vi "create scan vectr.vi"(2 "Table Control":string[][](table), 3 "waypoint mode?":bool=TRUE) -> (0 "Array 2":dbl[](array[numeric]), 1 "Array":dbl[](array[numeric]))   [LabVIEW 2020]
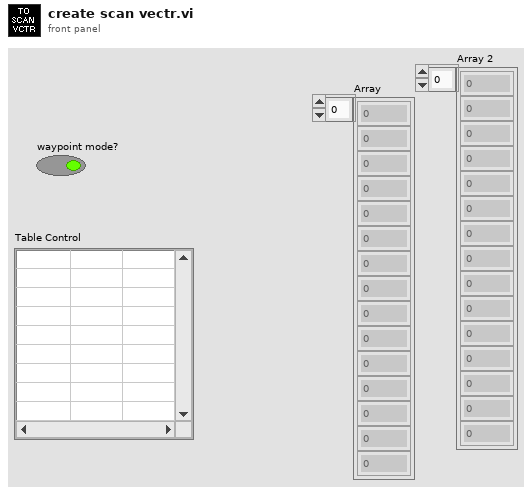
[diagram p1: front panel]
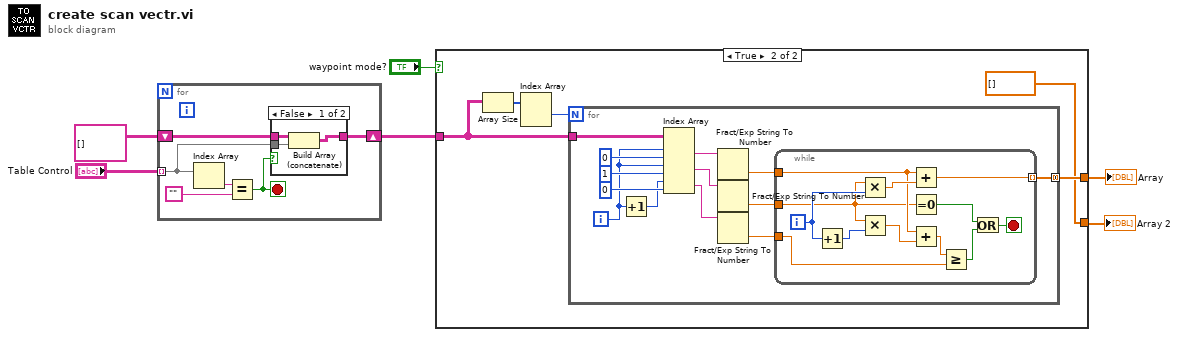
[diagram p0: block diagram]
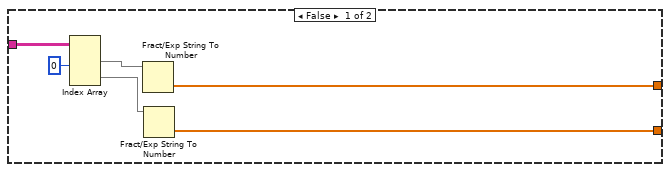
[diagram p2: hidden frame]
diagram:
  n1 = for {
    tunnel: "Table Control" -> [w8] mode=indexing
    shift-right: [w7] -> w3
    shift-left: string[][] [] ("t") -> [w10]
    stop <- w9 stop-if-true
    n2 = Index Array(array=w8) -> (element=w11:string)  [unwired: 1 in]
    n3 = Equal?(x=w11, y="") -> (x = y?=w9:bool)
    n4 = case shown="False" w9 {
      tunnel: w10 -> [w15 w16]
      tunnel: w8 -> [w14 _]
      tunnel: [w13 w16] -> w7
      frame False {
        n5 = Build Array (concatenate)(w15, w14) -> (w13:string[][])
      }
      frame True {
      }
    }
  }
  n6 = case shown="True" "waypoint mode?" {
    tunnel: [w20 w25] -> w4
    tunnel: w3 -> [w21 w24]
    tunnel: [w17 dbl[] []] -> w1
    frame False {
      n7 = Index Array(array=w21, index (col) #1=0 ("disabled index (col)")) -> (element #1=w22:string[], element #2=w18:string[])  [unwired: 3 in]
      n8 = Fract/Exp String To Number(string=w22) -> (number=w20:dbl[])  [unwired: 3 in, 1 out]
      n9 = Fract/Exp String To Number(string=w18) -> (number=w17:dbl[])  [unwired: 3 in, 1 out]
    }
    frame True {
      n10 = Array Size(array=w24) -> (size(s)=w27:i32[])
      n11 = Index Array(array=w27) -> (element #1=w26:i32)  [unwired: 2 in, 1 out]
      n12 = for {
        N: w26 -> [_]
        tunnel: w24 -> [w36]
        tunnel: [w28] -> w25 mode=concatenating
        i -> [w35]
        n13 = Increment(x=w35) -> (x+1=w38:i32)
        n14 = Index Array(array=w36, index (row) #1=w35, index (col) #1=0 ("disabled index (col)"), index (row) #2=w35, index (col) #2=1 ("disabled index (col)"), index (row) #3=w38, index (col) #3=0 ("disabled index (col)")) -> (element #1=w34:string, element #2=w33:string, element #3=w32:string)
        n15 = Fract/Exp String To Number(string=w34) -> (number=w31:dbl)  [unwired: 3 in, 1 out]
        n16 = Fract/Exp String To Number(string=w33) -> (number=w30:dbl)  [unwired: 3 in, 1 out]
        n17 = Fract/Exp String To Number(string=w32) -> (number=w29:dbl)  [unwired: 3 in, 1 out]
        n18 = while {
          tunnel: w31 -> [w47]
          tunnel: w30 -> [w44]
          tunnel: w29 -> [w45]
          tunnel: [w51] -> w28 mode=indexing
          i -> [w49]
          stop <- w41 stop-if-true
          n19 = Increment(x=w49) -> (x+1=w48:i32)
          n20 = Multiply(x=w44, y=w49) -> (x*y=w52:dbl)
          n21 = Multiply(x=w44, y=w48) -> (x*y=w50:dbl)
          n22 = Add(x=w47, y=w52) -> (x+y=w51:dbl)
          n23 = Equal To 0?(x=w44) -> (x = 0?=w43:bool)
          n24 = Add(x=w47, y=w50) -> (x+y=w46:dbl)
          n25 = Greater Or Equal?(x=w46, y=w45) -> (x >= y?=w42:bool)
          n26 = Or(x=w43, y=w42) -> (x .or. y?=w41:bool)
        }
      }
    }
  }
  "Array" <- w4
  "Array 2" <- w1
